vi "letterbox.vi"(7 "Size":T1={"x"=640, "y"=640}, 8 "error in (no error)":errorcluster, 10 "resized":refnum<class "Mat_8U.lvclass">, 11 "image":refnum<class "Mat_8U.lvclass">) -> (0 "error out":errorcluster, 3 "resized out":refnum<class "Mat_8U.lvclass">)   [LabVIEW 2023]
uses:
  <vilib>/addons/VIRobotics/opencv_yiku/Mat/Mat_8U/Mat_8U.lvclass
  C:/Program Files/National Instruments/LabVIEW 2023/vi.lib/addons/VIRobotics/opencv_yiku/Mat/Mat/Mat.lvclass
  <vilib>/addons/VIRobotics/opencv_yiku/ctls/Size.ctl
  <vilib>/addons/VIRobotics/opencv_yiku/Mat/Create_Mat_8U.vi
  <vilib>/addons/VIRobotics/opencv_yiku/Mat/Mat/Mat.lvclass
  <vilib>/addons/VIRobotics/opencv_yiku/opencv_yiku.lvlib
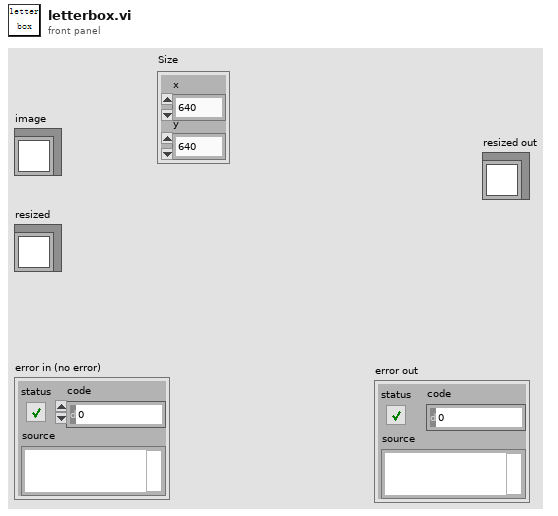
[diagram p1: front panel]
types:
  T1 = typedef "opencv_yiku.lvlib/Size.ctl" = cluster{"x":i32, "y":i32}
  T2 = cluster{"top":i32, "bottom":i32, "left":i32, "right":i32}
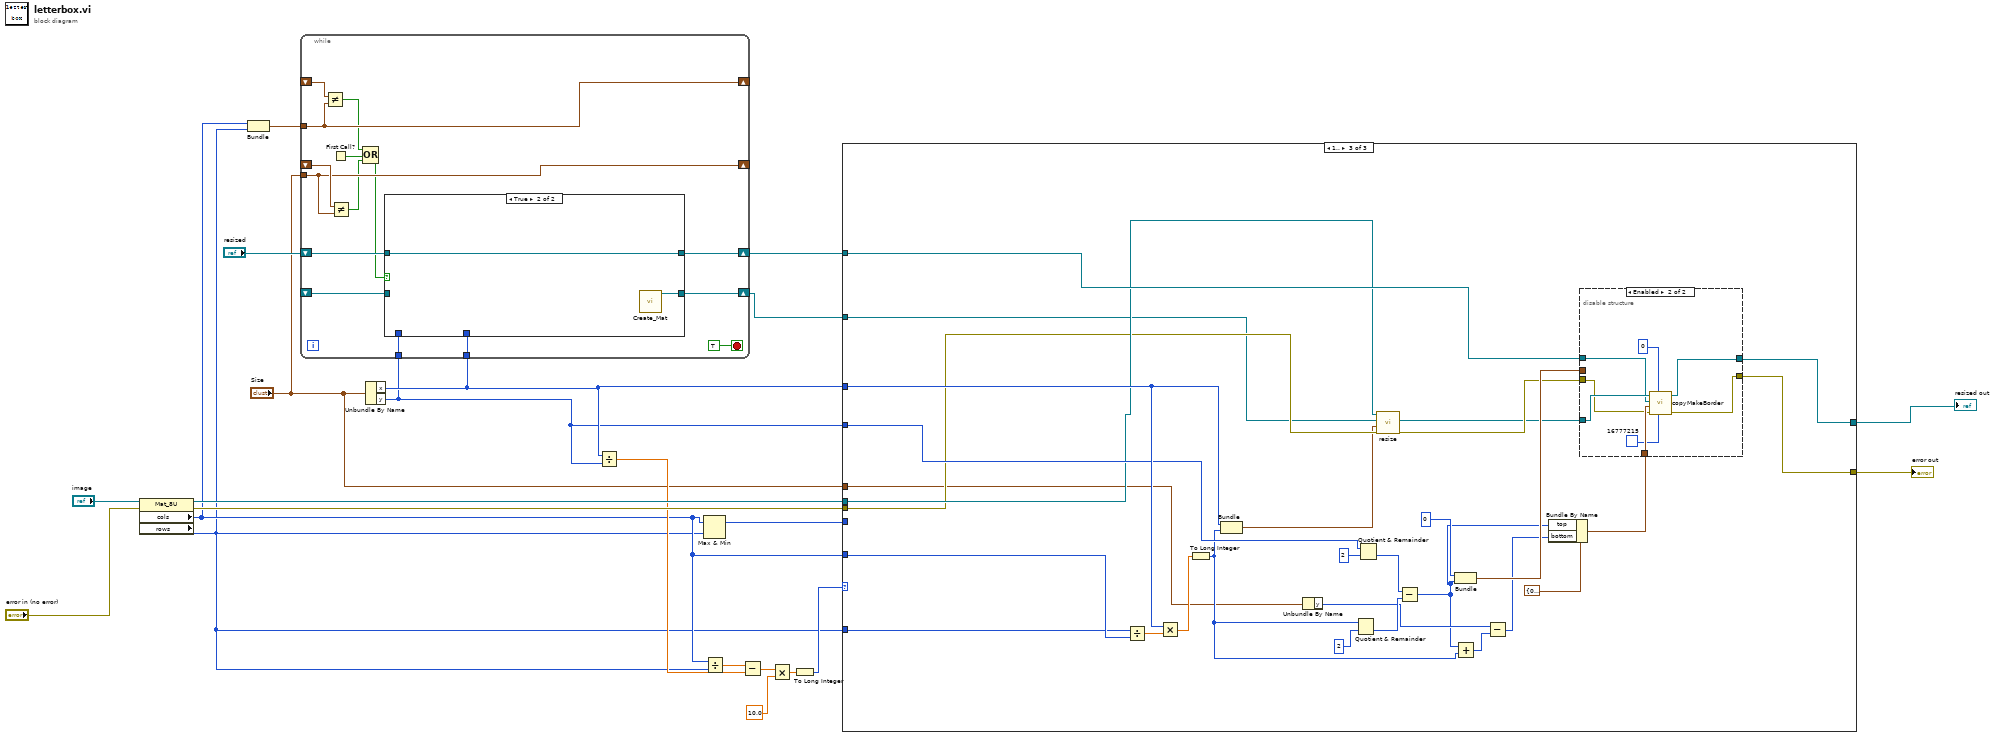
[diagram p0: block diagram]
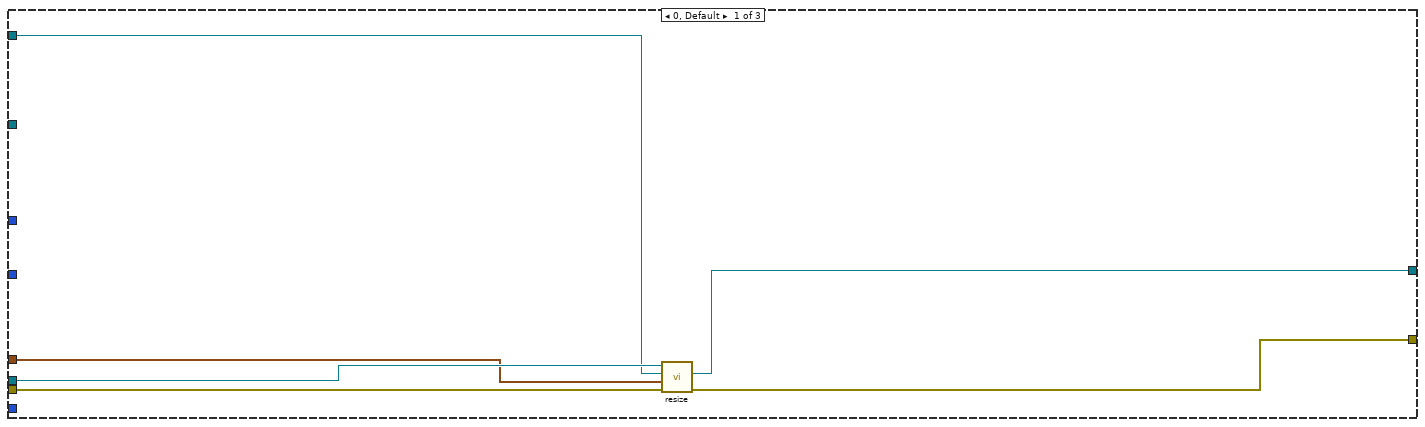
[diagram p3: hidden frame]
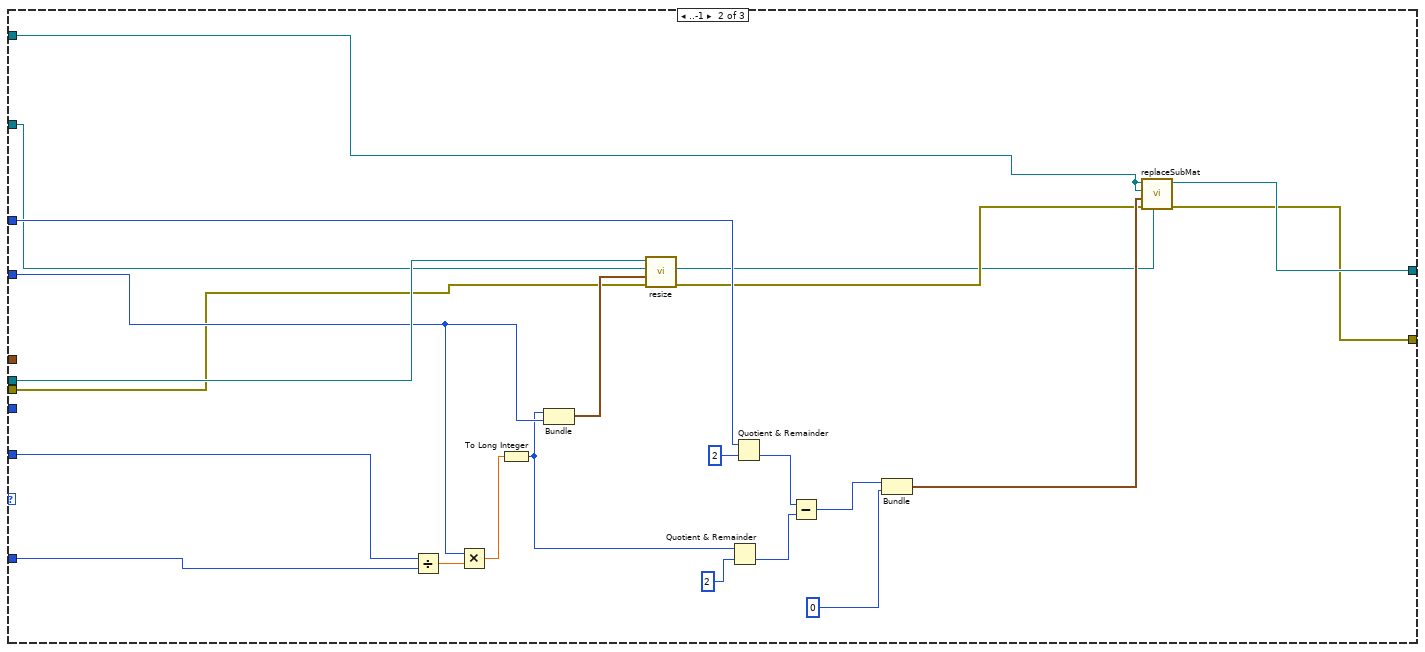
[diagram p4: hidden frame]
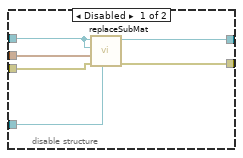
[diagram p5: hidden frame]
diagram:
  n1 = property class="Mat_8U"(reference="image", error in="error in (no error)") -> (reference out=w20:refnum<class "Mat_8U.lvclass">, error out=w18:errorcluster, "cols"=w4:i32, "rows"=w3:i32)
  n2 = Bundle("cols"=w4, "rows"=w3) -> (w2:cluster{"cols":i32, "rows":i32})  [unwired: 1 in]
  n3 = Unbundle By Name("Size") -> ("x"=w7:i32, "y"=w6:i32)
  n4 = while {
    tunnel: w7 -> [w35]
    tunnel: w6 -> [w34]
    shift-right: [w36] -> w8
    shift-left: "resized" -> [w37]
    tunnel: "Size" -> [w31]
    shift-right: [w31] -> _
    shift-left: _ -> [w32]
    tunnel: w2 -> [w29]
    shift-right: [w29] -> _
    shift-left: _ -> [w30]
    shift-right: [w24] -> w1
    shift-left: _ -> [w23]
    stop <- TRUE stop-if-true
    n5 = Not Equal?(x=w30, y=w29) -> (x != y?=w28:bool)
    n6 = First Call?() -> (First Call?: T/F=w26:bool)
    n7 = Not Equal?(x=w32, y=w31) -> (x != y?=w27:bool)
    n8 = Compound Arithmetic op=OR(w28, w26, w27) -> (w25:bool)
    n9 = case shown="True" w25 {
      tunnel: w37 -> [w39 w40]
      tunnel: [w39 w40] -> w36
      tunnel: w35 -> [_ _]
      tunnel: w34 -> [_ _]
      tunnel: [w38 w41] -> w24
      tunnel: w23 -> [w38 _]
      frame False {
      }
      frame True {
        n10 = call-poly <vilib>:"Create_Mat.vi"() -> ("Mat_8U_out"=w41:refnum<class "Mat_8U.lvclass">)  [unwired: 10 in, 1 out]
      }
    }
  }
  n11 = Divide(x=w7, y=w6) -> (x/y=w14:dbl)
  n12 = Max & Min(x=w4, y=w3) -> (max(x,y)=w21:i32)  [unwired: 1 out]
  n13 = Divide(x=w4, y=w3) -> (x/y=w15:dbl)
  n14 = Subtract(x=w15, y=w14) -> (x-y=w13:dbl)
  n15 = Multiply(x=w13, y=10.0) -> (x*y=w11:dbl)
  n16 = To Long Integer(number=w11) -> (32bit integer=w10:i32)
  n17 = case shown="1.." w10 {
    tunnel: w21 -> [_ _ _]
    tunnel: w4 -> [_ w69 w99]
    tunnel: w3 -> [_ w68 w98]
    tunnel: w20 -> [w47 w70 w83]
    tunnel: w18 -> [w45 w49 w82]
    tunnel: [w44 w48 w80] -> w17
    tunnel: w8 -> [w46 w53 w87]
    tunnel: [w43 w67 w97] -> w16
    tunnel: w7 -> [_ w66 w96]
    tunnel: w6 -> [_ w65 w95]
    tunnel: "Size" -> [w42 _ w76]
    tunnel: w1 -> [_ w50 w81]
    frame 0, Default {
      n18 = call <vilib>:"resize.vi"("error in (no error)"=w45, "Size"=w42, "dst"=w46, "src"=w47) -> ("error out"=w44:errorcluster, "dst out"=w43:refnum<class "Mat_8U.lvclass">)  [unwired: 5 in, 1 out]
    }
    frame ..-1 {
      n19 = Divide(x=w69, y=w68) -> (x/y=w64:dbl)
      n20 = Multiply(x=w65, y=w64) -> (x*y=w63:dbl)
      n21 = To Long Integer(number=w63) -> (32bit integer=w54:i32)
      n22 = Bundle(w54, "y"=w65) -> (w62:cluster{i32, "y":i32})  [unwired: 1 in]
      n23 = call <vilib>:"resize.vi"("error in (no error)"=w49, "Size"=w62, "dst"=w50, "src"=w70) -> ("error out"=w52:errorcluster, "dst out"=w51:refnum<class "Mat_8U.lvclass">)  [unwired: 5 in, 1 out]
      n24 = Quotient & Remainder(x=w54, y=2) -> (floor(x/y)=w58:i32)  [unwired: 1 out]
      n25 = Quotient & Remainder(x=w66, y=2) -> (floor(x/y)=w59:i32)  [unwired: 1 out]
      n26 = Subtract(x=w59, y=w58) -> (x-y=w56:i32)
      n27 = Bundle(w56, 0) -> (w57:cluster{i32, i32})  [unwired: 1 in]
      n28 = call <vilib>:"replaceSubMat.vi"("SubMat"=w51, "error in (no error)"=w52, "Point"=w57, "dst"=w53, "src in"=w53) -> ("error out"=w48:errorcluster, "dst out"=w67:refnum<class "Mat_8U.lvclass">)  [unwired: 5 in]
    }
    frame 1.. {
      n29 = Divide(x=w98, y=w99) -> (x/y=w94:dbl)
      n30 = Multiply(x=w96, y=w94) -> (x*y=w93:dbl)
      n31 = To Long Integer(number=w93) -> (32bit integer=w77:i32)
      n32 = Bundle("x"=w96, w77) -> (w78:cluster{"x":i32, i32})  [unwired: 1 in]
      n33 = Unbundle By Name(w76) -> ("y"=w75:i32)
      n34 = Quotient & Remainder(x=w77, y=2) -> (floor(x/y)=w89:i32)  [unwired: 1 out]
      n35 = Quotient & Remainder(x=w95, y=2) -> (floor(x/y)=w90:i32)  [unwired: 1 out]
      n36 = call <vilib>:"resize.vi"("error in (no error)"=w82, "Size"=w78, "dst"=w81, "src"=w83) -> ("error out"=w85:errorcluster, "dst out"=w84:refnum<class "Mat_8U.lvclass">)  [unwired: 5 in, 1 out]
      n37 = Subtract(x=w90, y=w89) -> (x-y=w72:i32)
      n38 = Bundle(0, w72) -> (w86:cluster{i32, i32})  [unwired: 1 in]
      n39 = Add(x=w72, y=w77) -> (x+y=w74:i32)
      n40 = Subtract(x=w75, y=w74) -> (x-y=w73:i32)
      n41 = Bundle By Name(cluster=T2 {"top"=0, "bottom"=0, "left"=0, "right"=0} ("border"), "top"=w72, "bottom"=w73) -> (w71:T2)
      n42 = disable-structure shown="Enabled" {
        disable-tunnel: [w105 w110] -> w97
        disable-tunnel: w87 -> [w104 w112]
        disable-tunnel: w86 -> [w103 _]
        disable-tunnel: w85 -> [w102 w107]
        disable-tunnel: w84 -> [w101 w113]
        disable-tunnel: [w100 w106] -> w80
        disable-tunnel: w71 -> [_ w109]
        frame Disabled {
          n43 = call <vilib>:"replaceSubMat.vi"("SubMat"=w101, "error in (no error)"=w102, "Point"=w103, "dst"=w104, "src in"=w104) -> ("error out"=w100:errorcluster, "dst out"=w105:refnum<class "Mat_8U.lvclass">)  [unwired: 5 in]
        }
        frame Enabled {
          n44 = call <vilib>:"copyMakeBorder.vi"("color"=u32 16777215, "type"=0, "error in (no error)"=w107, "border"=w109, "dst in"=w112, "Mat in"=w113) -> ("error out"=w106:errorcluster, "dst out"=w110:refnum<class "Mat_8U.lvclass">)  [unwired: 4 in]
        }
      }
    }
  }
  "resized out" <- w16
  "error out" <- w17
